vi "Get_center_pos.vi"() -> (1 "Position":dbl[](array[numeric]), 2 "flag":bool)   [LabVIEW 2012]
uses:
  <userlib>/dhd_sdk7/dhd_sdk7.lvlib
panel:
  out "Message":string
  out "error out":errorcluster
  in  "record":bool
  in  "stop":bool
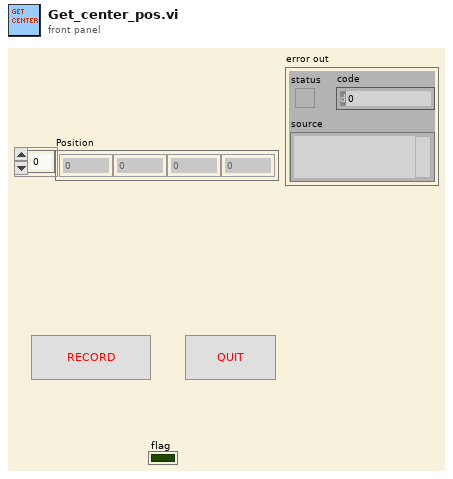
[diagram p1: front panel]
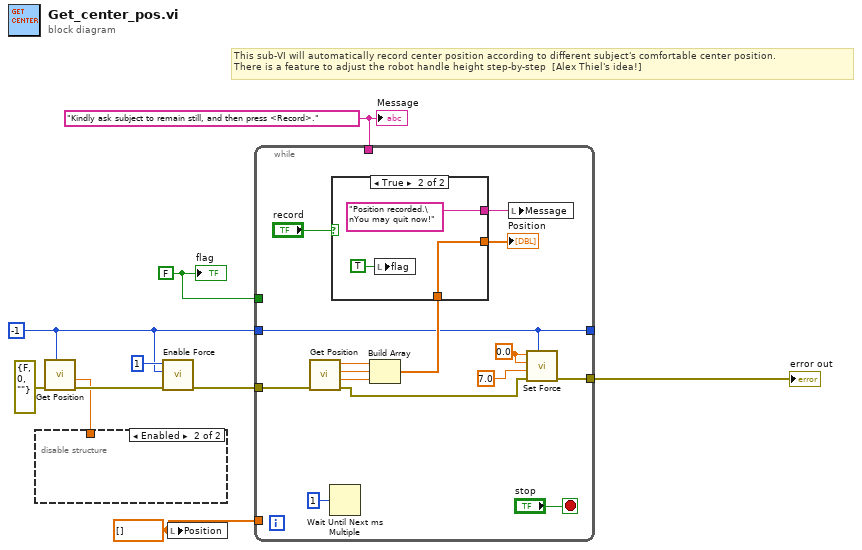
[diagram p0: block diagram]
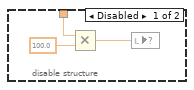
[diagram p2: hidden frame]
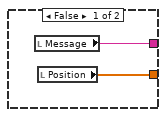
[diagram p3: hidden frame]
diagram:
  w1 = FALSE ("flag")
  w3 = "Kindly ask subject to remain still, and then press <Record>." ("source")
  w5 = -1
  w10 = dbl[] [] ("Array")
  # "This sub-VI will automatically record center position according to different subject's comfortable center position. \nThere is a feature to adjust the robot handle height step-by-step  [Alex Thiel's idea!]"
  n1 = call <userlib>:"Get Position.vi"("ID"=w5, "error in (no error)"=errorcluster {"status"=FALSE, "code"=0, "source"=""}) -> ("error out"=w7:errorcluster, "pz out"=w4:dbl)  [unwired: 5 in, 3 out]
  n2 = disable-structure shown="Enabled" {
    disable-tunnel: w4 -> [w13 _]
    frame Disabled {
      n3 = Multiply(x=w13, y=100.0) -> (x*y=w12:dbl)
      n4 = local write item#-1(w12) -> ()
    }
    frame Enabled {
    }
  }
  n5 = call <userlib>:"Enable Force.vi"("error in (no error)"=w7, "ID"=w5, "val"=u8 1) -> ("error out"=w9:errorcluster)  [unwired: 7 in, 1 out]
  n6 = local write "Position"(w10) -> ()
  n7 = while {
    tunnel: w10 -> [_]
    tunnel: [w20] -> w2
    tunnel: w9 -> [w19]
    tunnel: w5 -> [w18]
    tunnel: [w18] -> _
    tunnel: w3 -> [_]
    tunnel: w1 -> [_]
    stop <- "stop" stop-if-true
    w21 = 0.0 ("fx")
    n8 = call <userlib>:"Get Position.vi"("error in (no error)"=w19) -> ("error out"=w23:errorcluster, "pz out"=w14:dbl, "py out"=w15:dbl, "px out"=w16:dbl)  [unwired: 6 in, 1 out]
    n9 = Wait Until Next ms Multiple(millisecond multiple=u32 1) -> ()  [unwired: 1 out]
    n10 = Build Array(w16, w15, w14) -> (w24:dbl[])
    n11 = case shown="True" "record" {
      tunnel: [w30 w33] -> w25
      tunnel: w24 -> [_ w33]
      tunnel: [w29 "Position recorded.\nYou may quit now!" ("Message")] -> w17
      frame False {
        n12 = local read "Message"() -> (w29:string)
        n13 = local read "Position"() -> (w30:dbl[])
      }
      frame True {
        n14 = local write "flag"(TRUE ("flag")) -> ()
      }
    }
    "Position" <- w25
    n15 = local write "Message"(w17) -> ()
    n16 = call <userlib>:"Set Force.vi"("ID"=w18, "error in (no error)"=w23, "fz"=7.0, "fy"=w21, "fx"=w21) -> ("error out"=w20:errorcluster)  [unwired: 5 in, 1 out]
  }
  "error out" <- w2
  "Message" <- w3
  "flag" <- w1
